vi "optionsAcq_attenuator.vi"(6 "poll write":bool, 8 "error in (no error)":errorcluster, 9 "readWrite":enum16{"read", "write"}(ring), 10 "attenuator":bool, 11 "Thorlabs_OSA_64 in":refnum<class "OSA.lvclass">) -> (0 "error out":errorcluster, 1 "status":string, 2 "attenuator out":bool, 3 "Thorlabs_OSA_64 out":refnum<class "OSA.lvclass">, 4 "poll timeOut":bool)   [LabVIEW 2010, in "OSA.lvclass"]
uses:
  OSA.lvclass
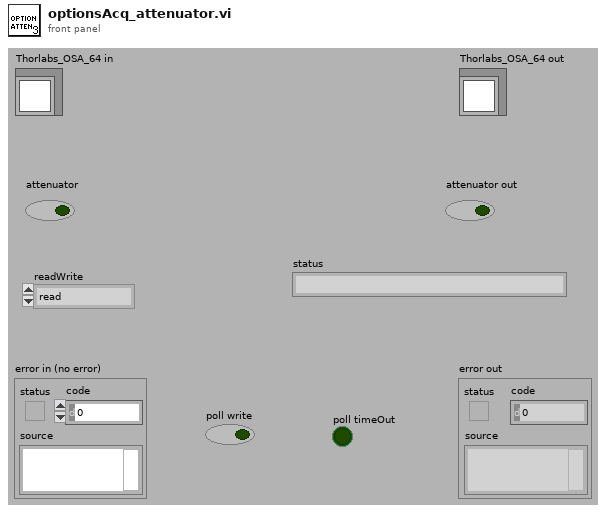
[diagram p1: front panel]
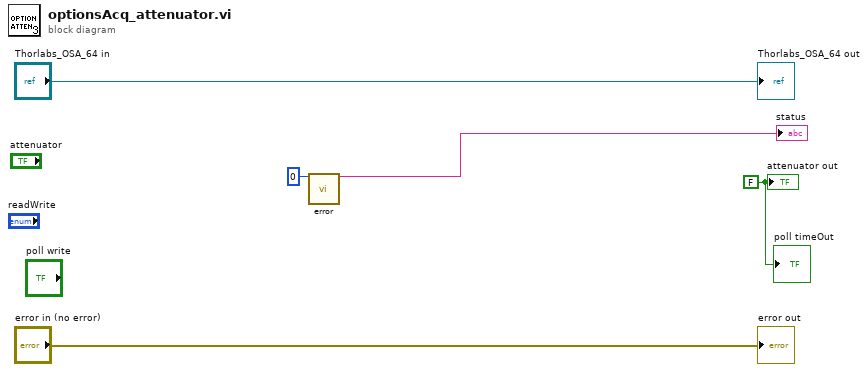
[diagram p0: block diagram]
diagram:
  w3 = FALSE ("attenuator out")
  n1 = call "error.vi"("result code"=0) -> ("status"=→"status":string)  [unwired: 16 in, 2 out]
  "error out" <- "error in (no error)"
  "Thorlabs_OSA_64 out" <- "Thorlabs_OSA_64 in"
  "poll timeOut" <- w3
  "attenuator out" <- w3
